vi "UI_Resize.vi"(8 "error in (no error)":errorcluster, 11 "LiveDatActor in":refnum<class "LiveDatActor.lvclass">) -> (0 "error out":errorcluster, 3 "LiveDatActor out":refnum<class "LiveDatActor.lvclass">)   [LabVIEW 2020, in "LiveDatActor.lvlib" / "LiveDatActor.lvclass"]
uses:
  LiveDatActor.lvclass
  LiveDatActor.lvclass/LiveDatActor.ctl
  support/UI_Actor.lvlibp/UI_Actor/UI_Actor.lvclass
panel:
  out ".not. x?":bool
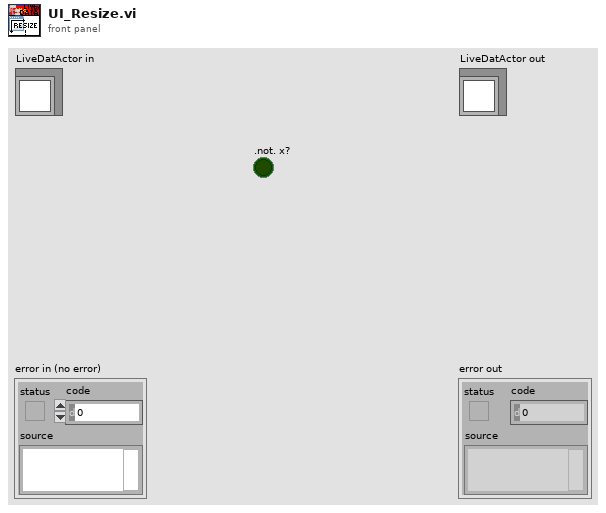
[diagram p1: front panel]
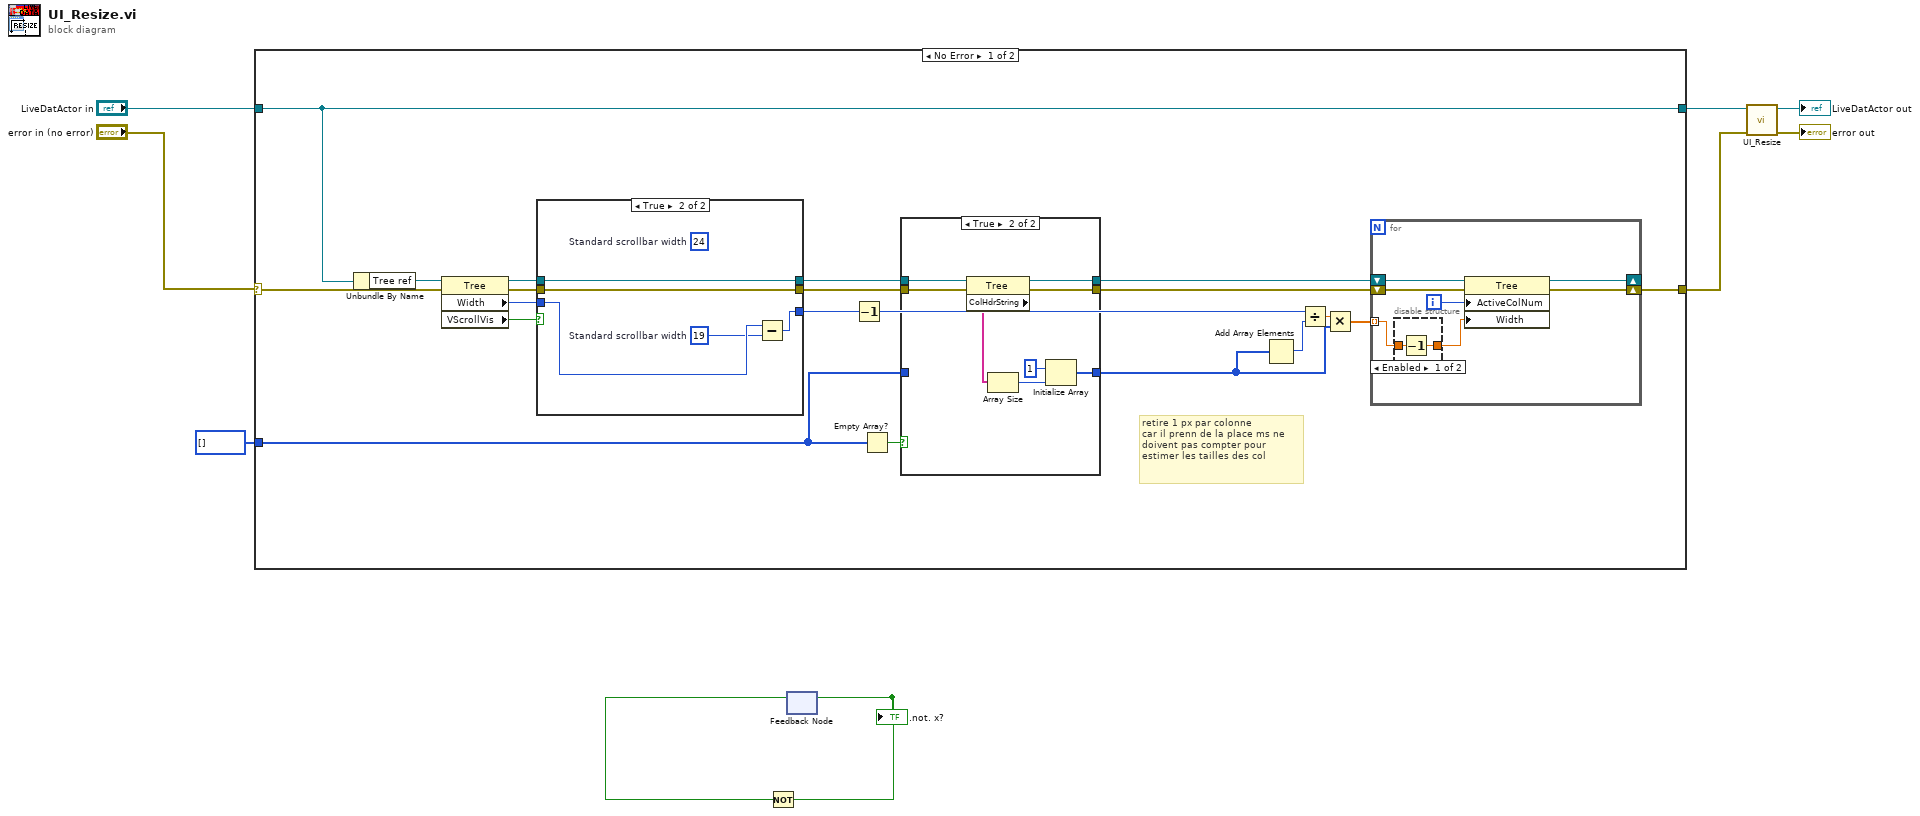
[diagram p0: block diagram]
diagram:
  n1 = case shown="No Error" "error in (no error)" {
    selector: "error in (no error)" -> [w12 w60]
    tunnel: [w10 w60] -> w5
    tunnel: [w14 w59] -> w6
    tunnel: "LiveDatActor in" -> [w14 w59]
    tunnel: u32[] [] ("Rapports des tailles") -> [w11 _]
    frame No Error {
      # "retire 1 px par colonne\ncar il prenn de la place ms ne doivent pas compter pour estimer les tailles des col"
      n2 = Unbundle By Name(w14) -> ("Tree ref"=w13:refnum<vi>)
      n3 = property on="Property Node" class="Tree"(reference=w13, error in=w12) -> (reference out=w19:refnum<vi>, error out=w20:errorcluster, "Width"=w18:u32, "VScrollVis"=w21:bool)
      n4 = case shown="True" w21 {
        tunnel: w18 -> [w41 w46]
        tunnel: [w41 w48] -> w27
        tunnel: w19 -> [w43 w45]
        tunnel: [w43 w45] -> w24
        tunnel: [w42 w47] -> w23
        tunnel: w20 -> [w42 w47]
        frame False {
        }
        frame True {
          (unwired) u32 24  # Standard scrollbar width
          w44 = u32 19  # Standard scrollbar width
          n5 = Subtract(x=w46, y=w44) -> (x-y=w48:u32)
        }
      }
      n6 = Decrement(x=w27) -> (x-1=w29:u32)
      n7 = Empty Array?(array=w11) -> (empty?=w22:bool)
      n8 = case shown="True" w22 {
        tunnel: [w32 w36] -> w28
        tunnel: w11 -> [w32 _]
        tunnel: w23 -> [w30 w40]
        tunnel: w24 -> [w31 w35]
        tunnel: [w31 w34] -> w25
        tunnel: [w30 w33] -> w26
        frame False {
        }
        frame True {
          n9 = property class="Tree"(reference=w35, error in=w40) -> (reference out=w34:refnum<vi>, error out=w33:errorcluster, "ColHdrString"=w37:string[])
          n10 = Array Size(array=w37) -> (size(s)=w38:i32)
          n11 = Initialize Array(u32 1 ("element"), w38) -> (w36:u32[])
        }
      }
      n12 = Add Array Elements(numeric array=w28) -> (sum=w17:u32)
      n13 = Divide(x=w29, y=w17) -> (x/y=w16:dbl)
      n14 = Multiply(x=w16, y=w28) -> (x*y=w15:dbl[])
      n15 = for {
        tunnel: w15 -> [w54] mode=indexing
        shift-right: [w51] -> w10
        shift-left: w26 -> [w52]
        shift-right: [w55] -> _
        shift-left: w25 -> [w53]
        i -> [w49]
        n16 = disable-structure shown="Enabled" {
          disable-tunnel: w54 -> [w57 w58]
          disable-tunnel: [w56 w58] -> w50
          frame Enabled {
            n17 = Decrement(x=w57) -> (x-1=w56:dbl)
          }
          frame Disabled {
          }
        }
        n18 = property on="Property Node" class="Tree"(reference=w53, error in=w52, "ActiveColNum"=w49, "Width"=w50) -> (reference out=w55:refnum<vi>, error out=w51:errorcluster)
      }
    }
    frame Error {
    }
  }
  n19 = feedback #1() -> (w2:bool)  [unwired: 1 in]
  n20 = Not(x=w2) -> (.not. x?=w1:bool)
  ".not. x?" <- w1
  n21 = feedback-in #1(w1) -> ()
  n22 = call-parent "UI_Resize.vi"("error in (no error)"=w5, "UI_Actor in"=w6) -> ("error out"=→"error out":errorcluster, "UI_Actor out"=→"LiveDatActor out":refnum<class "LiveDatActor.lvclass">)  [unwired: 8 in]
